vi "connection.vi"(8 "BAUD":i32, 10 "COM PORT":string, 11 "GPIB address":string) -> (3 "Connection":cluster{"queue out":refnum<queue>})   [LabVIEW 2019]
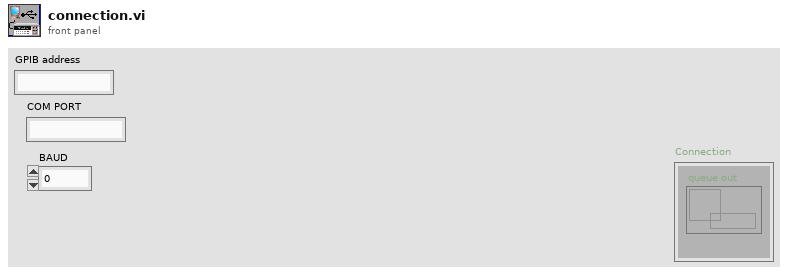
[diagram p1: front panel]
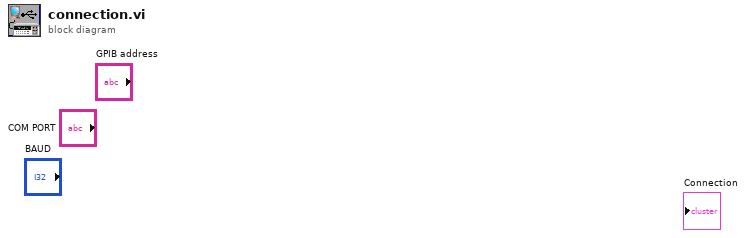
[diagram p0: block diagram]
diagram:
